vi "WaveformIO.vi"() -> ()   [LabVIEW 2015]
uses:
  <vilib>/Waveform/WDTFileIO.llb/ Write Waveform to File.vi
  <vilib>/measure/NI_MABase.lvlib
panel:
  out "Array":dbl[](array[numeric])
  out "Waveform Graph":waveform(dbl)(graph)
  in  "phase":dbl(knob) scale=0.0..10.0
  in  "amplitude":dbl(knob)=1.0 scale=0.0..10.0
  in  "frequency":dbl(knob)=10.0 scale=0.0..10.0
  in  "reset signal":bool
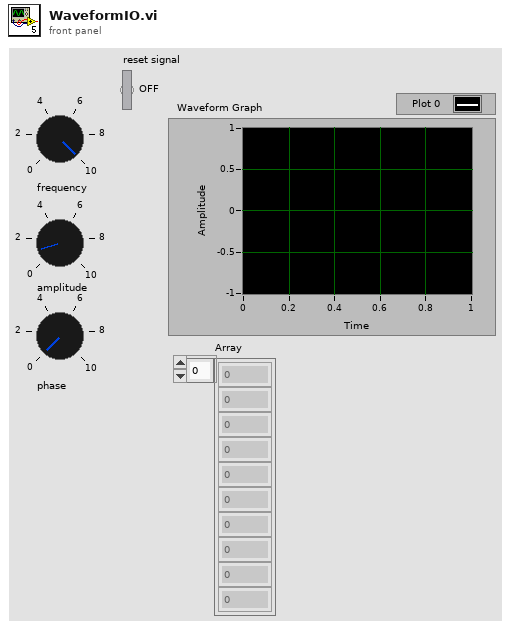
[diagram p1: front panel]
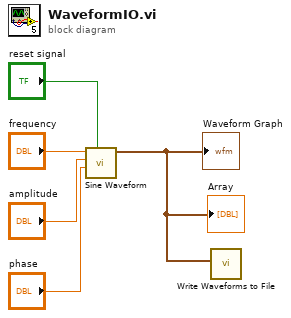
[diagram p0: block diagram]
diagram:
  n1 = call <vilib>:"Sine Waveform.vi"("reset signal"="reset signal", "phase"="phase", "amplitude"="amplitude", "frequency"="frequency") -> ("signal out"=w1:waveform(dbl))  [unwired: 6 in, 1 out]
  "Waveform Graph" <- w1
  "Array" <- w1
  n2 = call-poly <vilib>:"Write Waveforms to File.vi"("waveform"=w1) -> ()  [unwired: 9 in, 2 out]
